vi "Get Module Path from Identifier.vi"(8 "error in (no error)":errorcluster, 10 "Module identifier":string, 11 ".NET Refnum in":refnum<k24>) -> (0 "error out":errorcluster, 2 "Module path":string, 3 ".NET Refnum out":refnum<k24>)   [LabVIEW 2017, in "Routing and Faulting Scripting.lvlib"]
uses:
  Routing and Faulting Scripting.lvlib
  NationalInstruments.VeriStand.SystemStorage
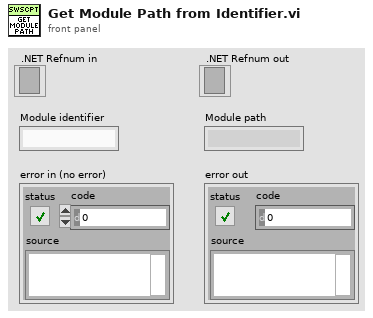
[diagram p1: front panel]
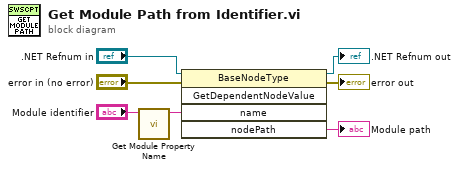
[diagram p0: block diagram]
diagram:
  n1 = call "Get Module Property Name.vi"("Module ID"="Module identifier") -> ("Module Property Name"=w4:string)  [unwired: 10 in]
  n2 = invoke class="BaseNodeType" method="GetDependentNodeValue"(reference=".NET Refnum in", error in="error in (no error)", "name"=w4) -> (reference out=→".NET Refnum out":refnum<k24>, error out=→"error out":errorcluster, "nodePath"=→"Module path":string)  [unwired: 2 in, 2 out]
